vi "Map - Reset.vi"(8 "error in (no error)":errorcluster, 11 "Map In":variant) -> (0 "error out":errorcluster, 3 "Map Out":variant)   [LabVIEW 2024]
doc: "Rests map and deletes all the nodes in <b>Map</b>."
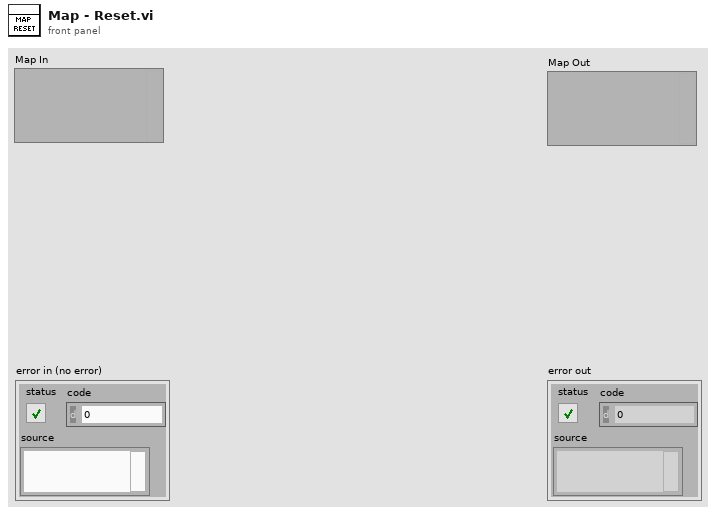
[diagram p1: front panel]
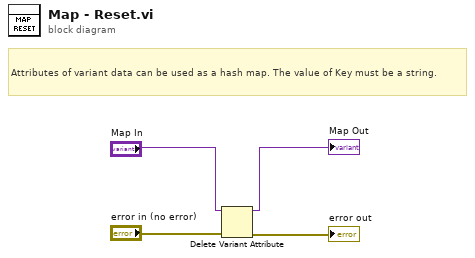
[diagram p0: block diagram]
diagram:
  # "Attributes of variant data can be used as a hash map. The value of Key must be a string."
  n1 = Delete Variant Attribute(4:"error in (no error)", 7:"Map In") -> (0:→"error out":errorcluster, 3:→"Map Out":variant)  [unwired: 1 in, 1 out]
